vi "Pre Launch Init.vi"(11 "Filter Config Display in":refnum<class "Filter Config Display.lvclass">) -> (0 "error out":errorcluster, 3 "Filter Config Display out":refnum<class "Filter Config Display.lvclass">)   [LabVIEW 2016, in "Assert API Components.lvlib" / "Assert Display.lvlib" / "Filter Config Display.lvlib" / "Filter Config Display.lvclass"]
doc: "(<B>Filename</B>: Actor Framework.lvlib:Actor.lvclass:Pre Launch Init.vi)\n\nDefines behavior that occurs after the Launch Nested Actor method is invoked but before the actor's Actor Core method begins running.\n\nBy default, this method does nothing. A descendant class may override it to define behavior."
uses:
  Filter Config Display.lvclass
  Assert API Components/Filter Configurations/Base Filter.lvclass
  Filter Config Display.lvclass/Filter Config Display.ctl
  Base UI Component/Base UI Component/Base UI Component.lvclass
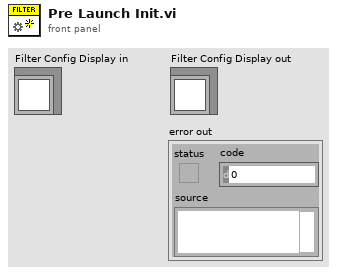
[diagram p1: front panel]
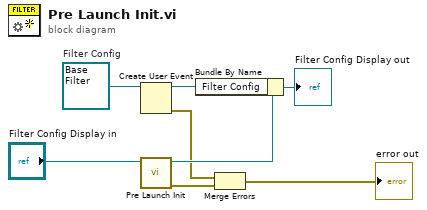
[diagram p0: block diagram]
diagram:
  w5 = refnum<class "Base Filter.lvclass"> refnum  # Filter Config
  n1 = Create User Event(user event datatype=w5) -> (user event=w3:refnum<user-event>, error out=w1:errorcluster)  [unwired: 1 in]
  n2 = call-parent "Pre Launch Init.vi"("Base UI Component in"="Filter Config Display in") -> ("error out"=w8:errorcluster, "Base UI Component out"=w7:refnum<class "Filter Config Display.lvclass">)  [unwired: 9 in]
  n3 = Bundle By Name(cluster=w7, "Filter Config"=w3) -> (→"Filter Config Display out":refnum<class "Filter Config Display.lvclass">)
  n4 = Merge Errors(w1, w8) -> (→"error out":errorcluster)
